vi "Unflatten Value.vi"(8 "error in (no error)":errorcluster, 10 "Value":string, 11 "Boolean in":refnum<class "Path.lvclass">) -> (0 "error out":errorcluster, 3 "Boolean out":refnum<class "Path.lvclass">)   [LabVIEW 2019, in "Path.lvclass"]
uses:
  <vilib>/gpm_packages/@cs/data-type-serializer/source/Path/Path.lvclass
  <vilib>/gpm_packages/@cs/data-type-serializer/source/Path/Path.lvclass/Path.ctl
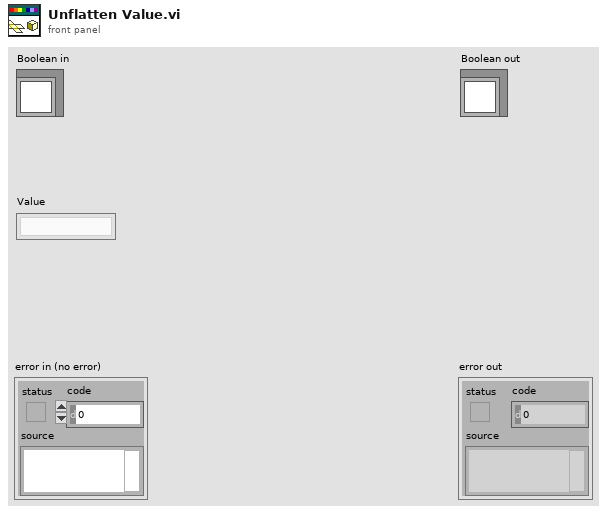
[diagram p1: front panel]
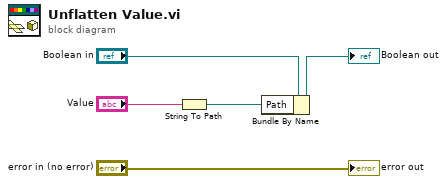
[diagram p0: block diagram]
diagram:
  n1 = String To Path(string="Value") -> (path=w1:path)
  n2 = Bundle By Name(cluster="Boolean in", "Path"=w1) -> (→"Boolean out":refnum<class "Path.lvclass">)
  "error out" <- "error in (no error)"
